vi "Instr_SetPrivateData.vi"(8 "error in (no error)":errorcluster, 11 "Switching in":refnum<class "Switching.lvclass">) -> (0 "error out":errorcluster, 3 "Switching out":refnum<class "Switching.lvclass">)   [LabVIEW 2013, in "Switching.lvclass"]
uses:
  Switching.lvclass
  InstrumentSetup.vi
  MUX_CommandsGlobal.vi
  Matrix_CommandsGlobal.vi
  InstrControl.lvclass
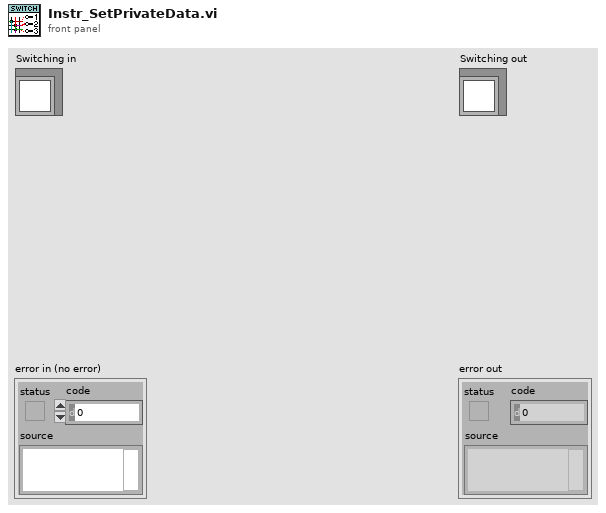
[diagram p1: front panel]
types:
  T1 = cluster{"GPIB address":string, "Matrix address":string, "Mux1 address":string, "Mux2 address":string, "Matrix used?":bool, "Switching":refnum<class "Switching.lvclass">, "Matrix X Channels":cluster{"Bias Supply / SMU LO":i32, "Bias Supply / SMU HI":i32, "CV Box LO":i32, "CV Box HI":i32, "CV Box LO IN":i32, "CV Box HI IN":i32, "Volt meter LO":i32, "Volt meter HI":i32, "Mux1 C1":i32, "Mux1 C2":i32, "Mux2 C1":i32, "Mux2 C2":i32}}
  T2 = cluster{"Matrix address":string, "Instrument name":string, "Instrument type":u16, "Command \"Matrix Reset\"":string, "Command \"Connect Matrix Channels\"":string, "Command \"Disconnect Matrix Channels\"":string}
  T3 = cluster{"Mux1 address":string, "Mux2 address":string, "Instrument name":string, "Instrument type":u16, "Command \"MUX Reset\"":string, "Command \"Select MUX Channel\"":string}
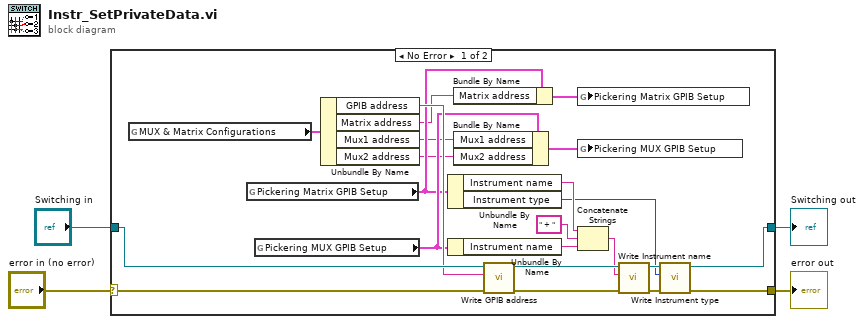
[diagram p0: block diagram]
diagram:
  n1 = case shown="No Error" "error in (no error)" {
    selector: "error in (no error)" -> [w21 w28]
    tunnel: [w13 w28] -> w3
    tunnel: "Switching in" -> [w20 w27]
    tunnel: [w12 w27] -> w1
    frame No Error {
      n2 = global read "InstrumentSetup.vi" "MUX & Matrix Configurations"() -> (w26:T1)
      n3 = global read "Matrix_CommandsGlobal.vi" "Pickering Matrix GPIB Setup"() -> (w10:T2)
      n4 = global read "MUX_CommandsGlobal.vi" "Pickering MUX GPIB Setup"() -> (w11:T3)
      n5 = Unbundle By Name(w26) -> ("GPIB address"=w19:string, "Matrix address"=w9:string, "Mux1 address"=w8:string, "Mux2 address"=w7:string)
      n6 = Unbundle By Name(w10) -> ("Instrument name"=w18:string, "Instrument type"=w14:u16)
      n7 = Unbundle By Name(w11) -> ("Instrument name"=w17:string)
      n8 = Bundle By Name(cluster=w10, "Matrix address"=w9) -> (w5:T2)
      n9 = Bundle By Name(cluster=w11, "Mux1 address"=w8, "Mux2 address"=w7) -> (w6:T3)
      n10 = call-dynamic "Write GPIB address.vi"("error in (no error)"=w21, "GPIB address"=w19, "InstControl in"=w20) -> ("error out"=w23:errorcluster, "InstControl out"=w25:refnum<class "Switching.lvclass">)  [unwired: 7 in]
      n11 = global write "Matrix_CommandsGlobal.vi" "Pickering Matrix GPIB Setup"(w5) -> ()
      n12 = global write "MUX_CommandsGlobal.vi" "Pickering MUX GPIB Setup"(w6) -> ()
      n13 = Concatenate Strings(w18, " + ", w17) -> (w15:string)
      n14 = call-dynamic "Write Instrument name.vi"("error in (no error)"=w23, "Instrument name"=w15, "InstControl in"=w25) -> ("error out"=w22:errorcluster, "InstControl out"=w24:refnum<class "Switching.lvclass">)  [unwired: 7 in]
      n15 = call-dynamic "Write Instrument type.vi"("error in (no error)"=w22, "Instrument type"=w14, "InstControl in"=w24) -> ("error out"=w13:errorcluster, "InstControl out"=w12:refnum<class "Switching.lvclass">)  [unwired: 7 in]
    }
    frame Error {
    }
  }
  "error out" <- w3
  "Switching out" <- w1
